vi "Choose View Type.vi"(8 "error in (no error)":errorcluster, 11 "Example Controller Actor in":refnum<class "Example Controller.lvclass">) -> (0 "error out":errorcluster, 3 "Example Controller Actor out":refnum<class "Example Controller.lvclass">)   [LabVIEW 2023, in "Example MVC Actors.lvlib" / "Example Controller.lvlib" / "Example Controller.lvclass"]
uses:
  Example Controller.lvclass
  Example View/Example View/Example View.lvclass
  Example Controller.lvclass/Example Controller.ctl
  properties/Write View Type.vi
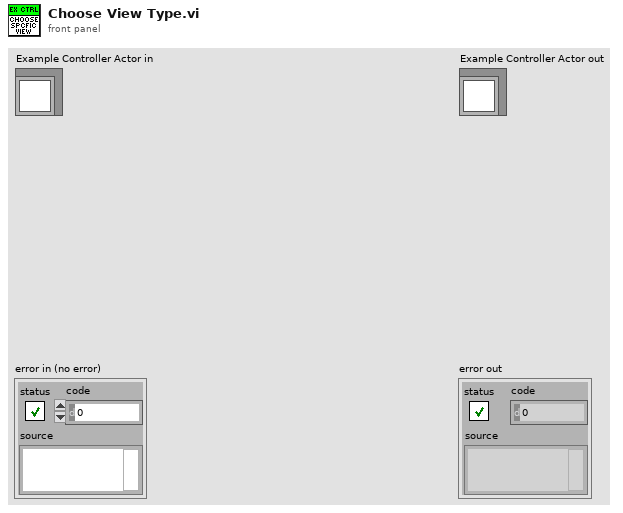
[diagram p1: front panel]
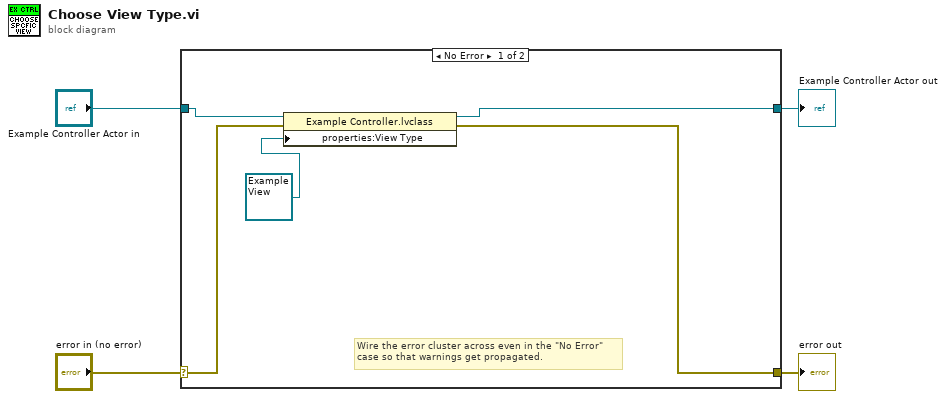
[diagram p0: block diagram]
diagram:
  n1 = case shown="No Error" "error in (no error)" {
    selector: "error in (no error)" -> [w7 w11]
    tunnel: [w5 w11] -> w3
    tunnel: [w8 w10] -> w1
    tunnel: "Example Controller Actor in" -> [w9 w10]
    frame No Error {
      # "Wire the error cluster across even in the \"No Error\"\ncase so that warnings get propagated."
      n2 = property class="Example Controller.lvclass"(reference=w9, error in=w7, "properties:View Type"=refnum<class "Example View.lvclass"> refnum ("Example View Actor.lvlib:Example View Actor.lvclass")) -> (reference out=w8:refnum<class "Example Controller.lvclass">, error out=w5:errorcluster)
    }
    frame Error {
    }
  }
  "error out" <- w3
  "Example Controller Actor out" <- w1
